vi "macro_TrajectoryGenerate.vi"   [LabVIEW 2019, in "Trajectory_Library.lvlib"]
uses:
  Trajectory_Library.lvlib
  Enum/TRAJECTORY_SPLINE_TYPE_ENUM.ctl
types:
  T1 = typedef "Trajectory_Library.lvlib/TRAJECTORY_SPLINE_TYPE_ENUM.ctl" = enum16{"Cubic", "Cubic With Weights", "Quintic", "Quintic With Weights"}
  T2 = typedef "Trajectory_Library.lvlib/TRAJ_CONFIG.ctl" = cluster{"MaxVelocity":dbl, "Max Acceleration":dbl, "StartVelocity":dbl, "End Velocity":dbl, "Reversed":bool, "Constraints":variant[]}
  T3 = typedef "Trajectory_Library.lvlib/WEIGHTED_WAYPOINT.ctl" = cluster{"TRANSLATION":T4, "ROTATION":T5, "SCALAR":dbl}
  T4 = typedef "Trajectory_Library.lvlib/TRANSLATION2D.ctl" = cluster{"X":dbl, "Y":dbl}
  T5 = typedef "Trajectory_Library.lvlib/ROTATION2D.ctl" = cluster{"VALUE":dbl, "COS":dbl, "SIN":dbl}
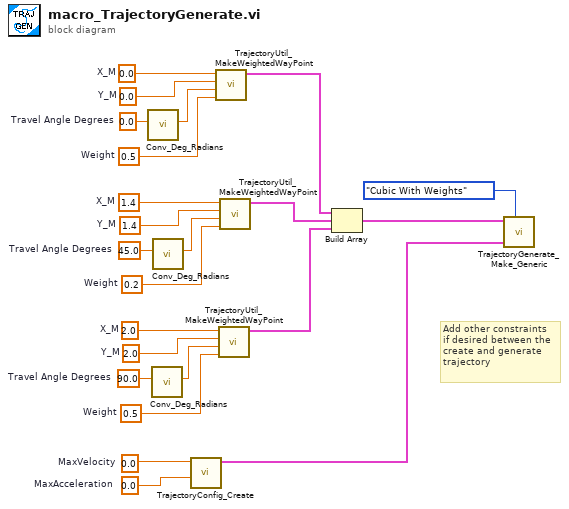
[diagram p0: block diagram]
diagram:
  w9 = 2.0  # X_M
  w10 = 2.0  # Y_M
  w2 = 90.0  # Travel Angle Degrees
  w11 = 0.5  # Weight
  w12 = 1.4  # X_M
  w13 = 1.4  # Y_M
  w4 = 45.0  # Travel Angle Degrees
  w14 = 0.2  # Weight
  w15 = 0.0  # X_M
  w16 = 0.0  # Y_M
  w5 = 0.0  # Travel Angle Degrees
  w17 = 0.5  # Weight
  w18 = 0.0  # MaxVelocity
  w19 = 0.0  # MaxAcceleration
  # "Add other constraints\nif desired between the\ncreate and generate\ntrajectory"
  n1 = call "Conv_Deg_Radians.vi"("Degress"=w5) -> ("Radians"=w6:dbl)  [unwired: 10 in]
  n2 = call "Conv_Deg_Radians.vi"("Degress"=w2) -> ("Radians"=w1:dbl)  [unwired: 10 in]
  n3 = call "Conv_Deg_Radians.vi"("Degress"=w4) -> ("Radians"=w3:dbl)  [unwired: 10 in]
  n4 = call "TrajectoryConfig_Create.vi"("MaxAcceleration"=w19, "MaxVelocity"=w18) -> ("TRAJECTORY_CONFIG"=w20:T2)  [unwired: 9 in]
  n5 = call "TrajectoryUtil_MakeWeightedWayPoint.vi"("Weight"=w17, "Travel Angle Radians"=w6, "Y_M"=w16, "X_M"=w15) -> ("WEIGHTED_WAYPOINT"=w23:T3)  [unwired: 7 in]
  n6 = call "TrajectoryUtil_MakeWeightedWayPoint.vi"("Weight"=w11, "Travel Angle Radians"=w1, "Y_M"=w10, "X_M"=w9) -> ("WEIGHTED_WAYPOINT"=w7:T3)  [unwired: 7 in]
  n7 = call "TrajectoryUtil_MakeWeightedWayPoint.vi"("Weight"=w14, "Travel Angle Radians"=w3, "Y_M"=w13, "X_M"=w12) -> ("WEIGHTED_WAYPOINT"=w8:T3)  [unwired: 7 in]
  n8 = Build Array(w23, w8, w7) -> (w22:T3[])
  n9 = call "TrajectoryGenerate_Make_Generic.vi"("Spline Type"=TRAJECTORY_SPLINE_TYPE_ENUM."Cubic With Weights", "traj_config"=w20, "WeightedWayPoints"=w22) -> ()  [unwired: 7 in, 2 out]
